vi "PPMS.Get Chamber.vi"(8 "error in (no error)":errorcluster, 11 "instrument.PPMS":refnum<class "instrument.PPMS.lvclass">) -> (0 "error out":errorcluster, 2 "Status String":string, 3 "instrument.PPMS out":refnum<class "instrument.PPMS.lvclass">)   [LabVIEW 2019, in "instrument.PPMS.lvclass"]
uses:
  instrument.PPMS.lvclass
  instrument.PPMS.lvclass/instrument.PPMS.ctl
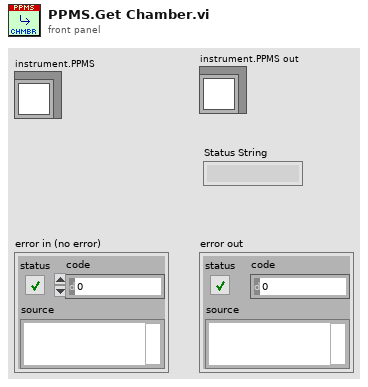
[diagram p1: front panel]
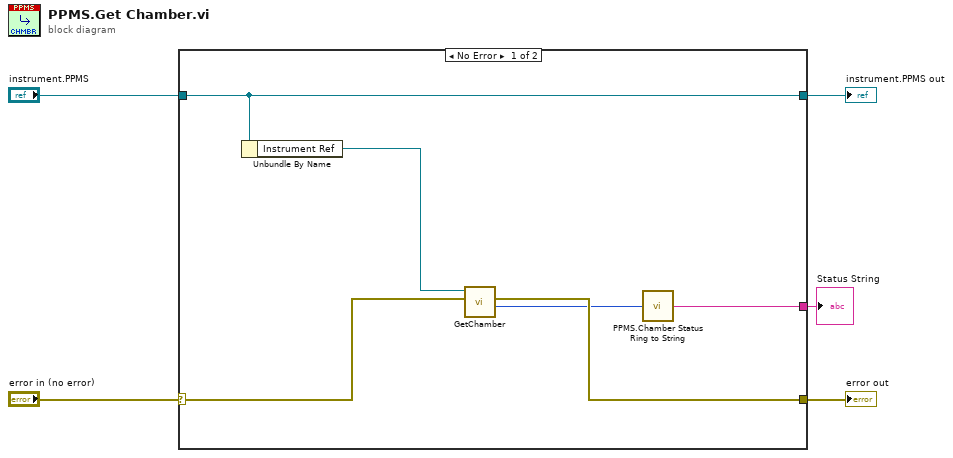
[diagram p0: block diagram]
diagram:
  n1 = case shown="No Error" "error in (no error)" {
    selector: "error in (no error)" -> [w9 w13]
    tunnel: [w8 w13] -> w5
    tunnel: "instrument.PPMS" -> [w11 w12]
    tunnel: [w11 w12] -> w2
    tunnel: [w6 _] -> w1
    frame No Error {
      n2 = Unbundle By Name(w11) -> ("Instrument Ref"=w10:refnum<k24>)
      n3 = call "GetChamber.vi"("error in (no error)"=w9, "Instrument Ref In"=w10) -> ("Chamber\nStatus"=w7:i32, "error out"=w8:errorcluster)  [unwired: 2 in, 2 out]
      n4 = call "PPMS.Chamber Status Ring to String.vi"("Chamber Status"=w7) -> ("Status String"=w6:string)
    }
    frame Error {
    }
  }
  "error out" <- w5
  "instrument.PPMS out" <- w2
  "Status String" <- w1
